vi "CAN test do RIO 1.vi"() -> ()   [LabVIEW 2014]
doc: "This example demonstrates frame streaming output using an NI-Embedded CAN for RIO interface. \n\nThis example can run against any input example, assuming you have a properly terminated CAN cable connected to two CAN ports."
uses:
  <vilib>/RioEmbeddedCAN/RioEmbeddedCAN.llb/CANFrameControl.ctl
  <vilib>/Platform/TimedLoop/XDataNode/timing_clust.ctl
  <vilib>/Platform/TimedLoop/XDataNode/nitl_modes.ctl
  <vilib>/Platform/TimedLoop/XDataNode/wakeup.ctl
  <vilib>/Platform/TimedLoop/XDataNode/XDataNode.xnode
  <vilib>/Platform/TimedLoop/XDataNode/XDNodeRunTimeDep.lvlib
panel:
  in  "odczyt":bool
  out "ilosc mesagy":dbl
  out "okres":dbl
  in  "ramki":bool
  in  "stop 2":bool
  in  "odczyt 2":bool=TRUE
  out "Frames 2":string[][](table) caption="Frames"
  in  "Number of Frames to Display 2":i32=15
  in  "Hexadecimal? 2":bool
  out "Numeric":i32
  in  "CAN frame 2":T1={"identifier"=2, "extended?"=FALSE, "type"=0, "payload"=[1, 2, 3, 4, 5, 6, 7, 8]} {"type" items=["CAN Data", "CAN Remote"]; "identifier" format="%.0x"}
  in  "Stop Button":bool
  in  "receive queue size":u32=50
  in  "baud rate":u32=500000
  in  "interface index":u32
  # "Interface Configuration"
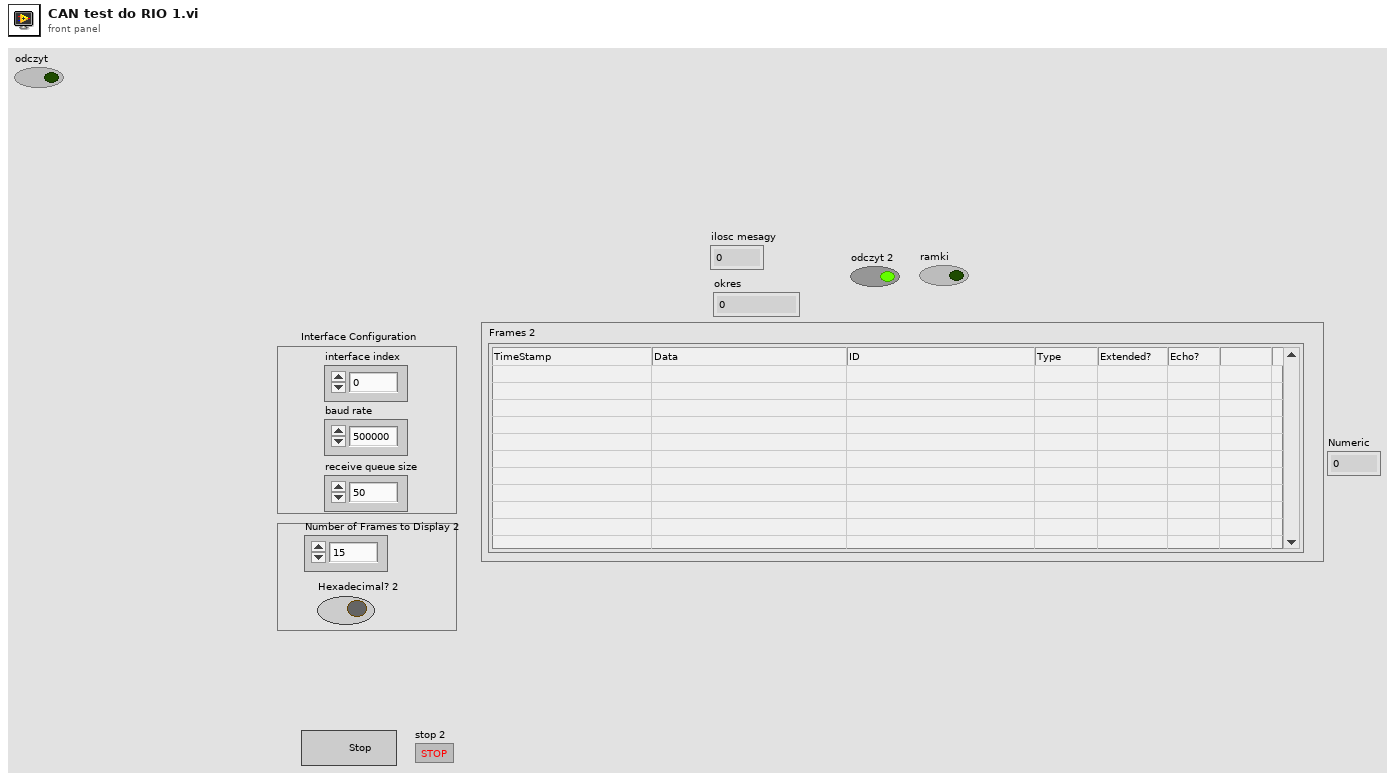
[diagram p1: front panel]
types:
  T1 = typedef "CANFrameControl.ctl" = cluster{"identifier":u32, "extended?":bool, "type":u8, "payload":u8[]}
  T2 = typedef "XDNodeRunTimeDep.lvlib/timing_clust.ctl" = cluster{"Expected End [f-1]":u64, "Actual End [f-1]":u64, "Finished Late? [f-1]":bool, "Expected End [i-1]":u64, "Actual End [i-1]":u64, "Finished Late? [i-1]":bool, "Expected Start [i]":u64, "Actual Start [i]":u64, "Expected Start [f]":u64, "Actual Start [f]":u64, "Source Name":string, "Structure Name":string, "Period":i64, "Deadline":i64, "Offset":i64, "Start":i64, "Priority":i32, "Timeout":i32, "Mode":T3, "Wakeup Reason":T4, "Error":errorcluster, "Source Type":string, "Secondary Source Type":string, "Global End Time":u64, "Global Start Time":u64, "Frame Duration":u64, "Iteration Duration":u64, "Assigned CPU":i32, "I/O Scan Engine Mode":u32}
  T3 = typedef "XDNodeRunTimeDep.lvlib/nitl_modes.ctl" = enum32{"No Change", "Process missed periods, maintain original phase", "Discard missed periods, maintain original phase", "Process missed periods, ignore original phase", "Discard missed periods, ignore original phase"}
  T4 = typedef "XDNodeRunTimeDep.lvlib/wakeup.ctl" = enum32{"Normal", "Aborted", "Asynchronous wakeup", "Timing source error", "Timed loop error", "Timeout"}
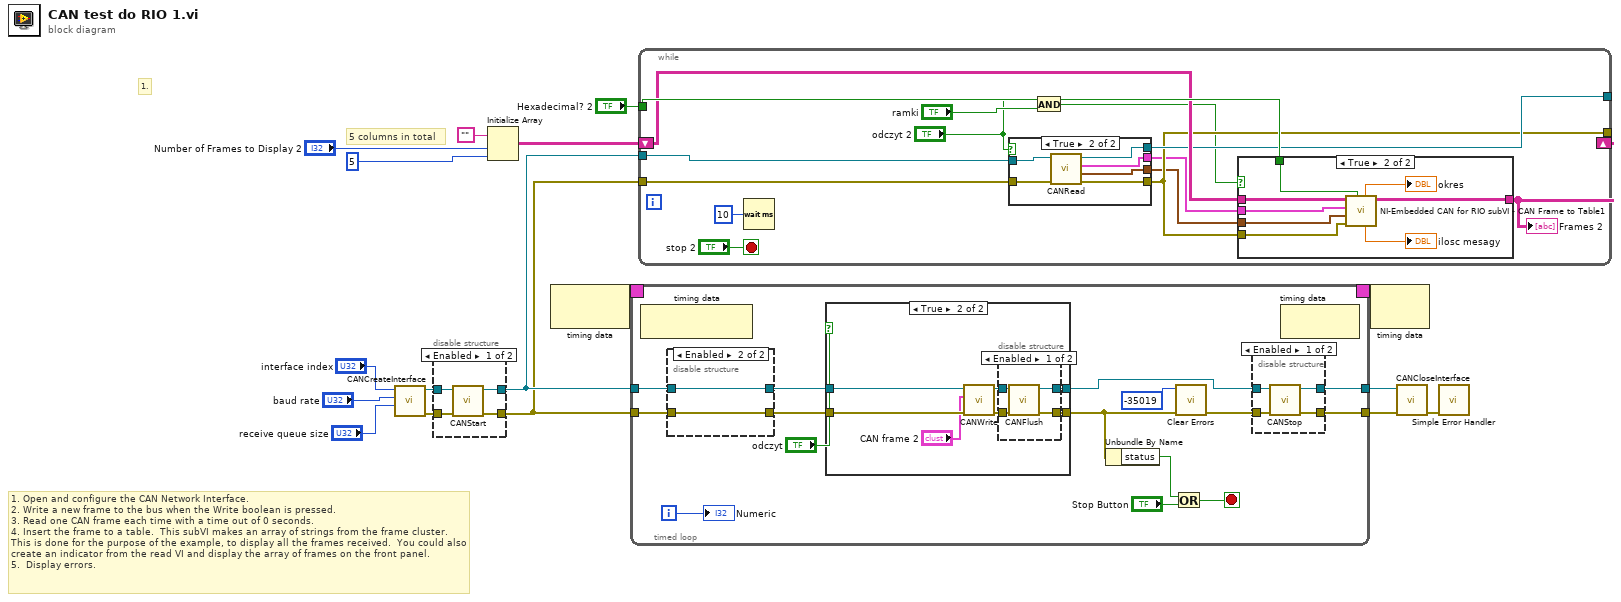
[diagram p0: block diagram]
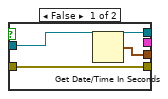
[diagram p3: hidden frame]
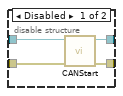
[diagram p5: hidden frame]
diagram:
  # "1. Open and configure the CAN Network Interface.\n2. Write a new frame to the bus when the Write boolean is pressed.\n3. Read one CAN frame each time with a time out of 0 seconds.\n4. Insert the frame to a table.  This subVI makes an array of strings from the frame cluster.  This is done for the purpose of the example, to display all the frames received.  You could also create an indicator from the read VI and display the array of frames on the front panel. \n5.  Display errors."
  # "5 columns in total"
  # "1."
  n1 = call <vilib>:"CANCreateInterface.vi"("receive queue size (5)"="receive queue size", "baud rate (125000 bps)"="baud rate", "interface index"="interface index") -> ("error out"=w8:errorcluster, "interface object out"=w9:refnum<k20>)  [unwired: 7 in]
  n2 = disable-structure shown="Enabled" {
    disable-tunnel: w9 -> [w21 w23]
    disable-tunnel: [w20 w23] -> w7
    disable-tunnel: w8 -> [w19 w22]
    disable-tunnel: [w18 w22] -> w6
    frame Enabled {
      n3 = call <vilib>:"CANStart.vi"("error in (no error)"=w19, "interface object in"=w21) -> ("error out"=w18:errorcluster, "interface object out"=w20:refnum<k20>)  [unwired: 8 in]
    }
    frame Disabled {
    }
  }
  n4 = Initialize Array("" ("Empty String Constant"), "Number of Frames to Display 2", 5 ("dimension size")) -> (w2:string[][])
  n5 = node-c288 ("Input Node")() -> (w17:T2)  [unwired: 1 in]
  n6 = timed-loop "Timed Loop" {
    timing: w17 -> [_]
    timing-out: [_] -> w16
    tunnel: w7 -> [w31]
    tunnel: w6 -> [w30]
    tunnel: [w34] -> w14
    tunnel: [w32] -> w13
    i -> [w29]
    stop <- w37 stop-if-true
    n7 = node-c288 ("Output Node")() -> ()  [unwired: 1 in, 1 out]
    n8 = disable-structure shown="Enabled" {
      disable-tunnel: w31 -> [w42 w43]
      disable-tunnel: [w41 w43] -> w26
      disable-tunnel: w30 -> [w40 w44]
      disable-tunnel: [w39 w44] -> w25
      frame Disabled {
        n9 = call <vilib>:"CANStart.vi"("error in (no error)"=w40, "interface object in"=w42) -> ("error out"=w39:errorcluster, "interface object out"=w41:refnum<k20>)  [unwired: 8 in]
      }
      frame Enabled {
      }
    }
    n10 = case shown="True" "odczyt" {
      tunnel: w25 -> [w52 w56]
      tunnel: [w51 w55] -> w27
      tunnel: [w52 w54] -> w28
      tunnel: w26 -> [w51 w57]
      frame False {
      }
      frame True {
        n11 = call <vilib>:"CANWrite.vi"("error in (no error)"=w56, "CAN frame"="CAN frame 2", "interface object in"=w57) -> ("error out"=w58:errorcluster, "interface object out"=w59:refnum<k20>)  [unwired: 7 in]
        n12 = disable-structure shown="Enabled" {
          disable-tunnel: w59 -> [w63 w65]
          disable-tunnel: w58 -> [w62 w64]
          disable-tunnel: [w61 w65] -> w55
          disable-tunnel: [w60 w64] -> w54
          frame Enabled {
            n13 = call <vilib>:"CANFlush.vi"("error in (no error)"=w62, "interface object in"=w63) -> ("error out"=w60:errorcluster, "interface object out"=w61:refnum<k20>)  [unwired: 8 in]
          }
          frame Disabled {
          }
        }
      }
    }
    n14 = Unbundle By Name(w28) -> ("status"=w38:bool)
    n15 = Or(x=w38, y="Stop Button") -> (x .or. y?=w37:bool)
    n16 = call <vilib>:"Clear Errors.vi"("error in (no error)"=w28, "specific error code to clear (0: all)"=-35019) -> ("error out"=w33:errorcluster)  [unwired: 4 in, 1 out]
    n17 = disable-structure shown="Enabled" {
      disable-tunnel: w27 -> [w48 w50]
      disable-tunnel: [w47 w50] -> w34
      disable-tunnel: w33 -> [w46 w49]
      disable-tunnel: [w45 w49] -> w32
      frame Enabled {
        n18 = call <vilib>:"CANStop.vi"("error in (no error)"=w46, "interface object in"=w48) -> ("error out"=w45:errorcluster, "interface object out"=w47:refnum<k20>)  [unwired: 8 in]
      }
      frame Disabled {
      }
    }
    n19 = node-c288 ("Input Node")() -> ()  [unwired: 1 in, 1 out]
    "Numeric" <- w29
  }
  n20 = while {
    tunnel: w7 -> [w69]
    tunnel: w6 -> [w68]
    shift-right: [w79] -> _
    shift-left: w2 -> [w80]
    tunnel: "Hexadecimal? 2" -> [w81]
    tunnel: [w76] -> _
    tunnel: [w77] -> _
    stop <- "stop 2" stop-if-true
    n21 = Wait (ms)(milliseconds to wait=u32 10) -> ()  [unwired: 1 out]
    n22 = case shown="True" "odczyt 2" {
      tunnel: w69 -> [w92 w99]
      tunnel: w68 -> [w93 w98]
      tunnel: [w91 w97] -> w70
      tunnel: [w93 w96] -> w76
      tunnel: [_ w95] -> w74
      tunnel: [w92 w94] -> w77
      frame False {
        n23 = Get Date/Time In Seconds() -> (seconds since 1Jan1904=w91:timestamp)
      }
      frame True {
        n24 = call <vilib>:"CANRead.vi"("error in (no error)"=w98, "interface object in"=w99) -> ("error out"=w96:errorcluster, "timestamp"=w97:timestamp, "CAN frame"=w95:T1, "interface object out"=w94:refnum<k20>)  [unwired: 6 in]
      }
    }
    n25 = And(x="odczyt 2", y="ramki") -> (x .and. y?=w73:bool)
    n26 = case shown="True" w73 {
      tunnel: w70 -> [_ w90]
      tunnel: w81 -> [_ w89]
      tunnel: w80 -> [w82 w88]
      tunnel: [w82 w87] -> w79
      tunnel: w76 -> [_ w86]
      tunnel: w74 -> [_ w85]
      frame False {
      }
      frame True {
        n27 = call "NI-Embedded CAN for RIO subVI - CAN Frame to Table1.vi"("Hexadecimal?"=w89, "error in (no error)"=w86, "timestamp"=w90, "CAN frame"=w85, "Input Array"=w88) -> ("Output Array"=w87:string[][], "ilosc mesagy"=→"ilosc mesagy":dbl, "okres 100"=→"okres":dbl)  [unwired: 2 in, 2 out]
      }
    }
    "Frames 2" <- w79
  }
  n28 = node-c288 ("Output Node")(w16) -> ()  [unwired: 1 out]
  n29 = call <vilib>:"CANCloseInterface.vi"("error in (no error)"=w13, "interface object in"=w14) -> ("error out"=w15:errorcluster)  [unwired: 9 in]
  n30 = call <vilib>:"Simple Error Handler.vi"("error in (no error)"=w15) -> ()  [unwired: 4 in, 5 out]
